vi "Variant-with-Array-Data-Type_to_String.vi"(8 "error in (no error)":errorcluster, 11 "variant":variant) -> (0 "error out":errorcluster, 3 "string":string)   [LabVIEW 2013]
doc: "Converts a variant, which contains an array element of almost any type, to a concatenated string where each value is separated by a space."
uses:
  <vilib>/Utility/VariantDataType/VariantType.lvlib
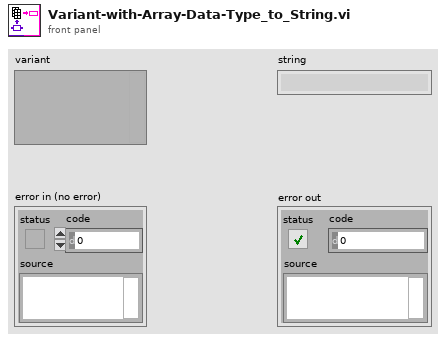
[diagram p1: front panel]
types:
  T1 = typedef "VariantType.lvlib/Type.ctl" = enum8{"Invalid Type", "Void", "I8", "I16", "I32", "I64", "U8", "U16", "U32", "U64", "Single Float", "Double Float", "Extended Float", "Single Complex", "Double Complex", "Extended Complex", "Enum U8", "Enum U16", "Enum U32", "Enum U64", "Single Float With Unit", "Double Float With Unit", "Extended Float With Unit", "Single Complex with Unit", "Double Complex with Unit", "Extended Complex with Unit", "Boolean", "String", "Path", "Picture", "Tag", "Array", "Cluster", "Variant", "LV Variant", "Waveform", "Timestamp", "Digital Waveform", "Digital Data", "ExpressData", "Refnum", "External Data", "VI", "Poly VI", "LabVIEW Class Instance", "Fixed Point"}
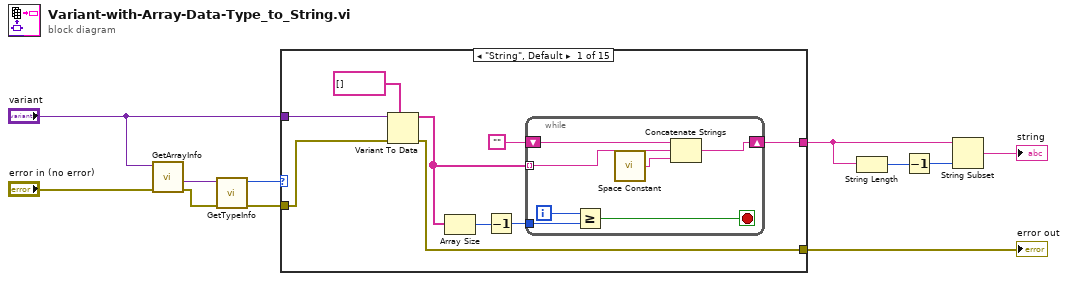
[diagram p0: block diagram]
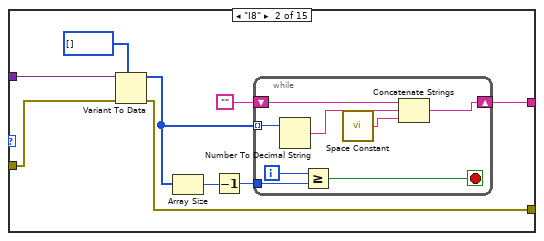
[diagram p2: hidden frame]
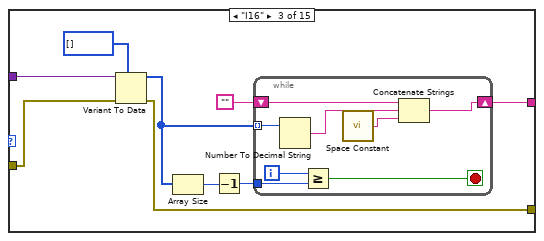
[diagram p3: hidden frame]
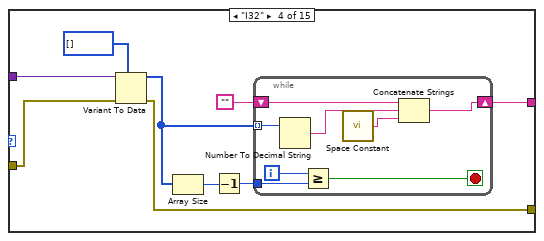
[diagram p4: hidden frame]
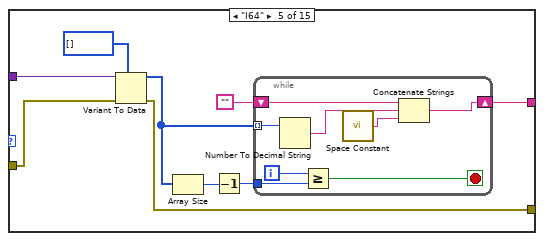
[diagram p5: hidden frame]
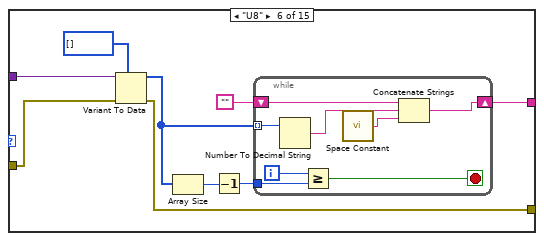
[diagram p6: hidden frame]
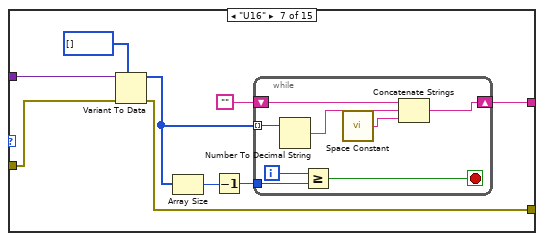
[diagram p7: hidden frame]
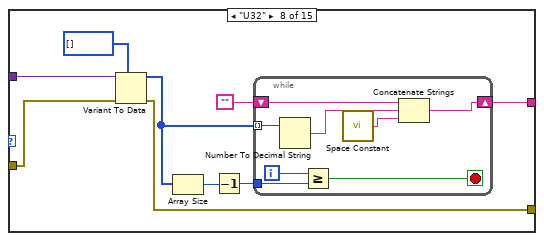
[diagram p8: hidden frame]
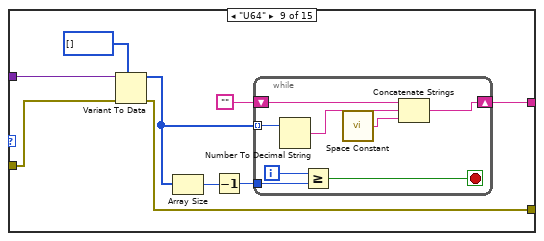
[diagram p9: hidden frame]
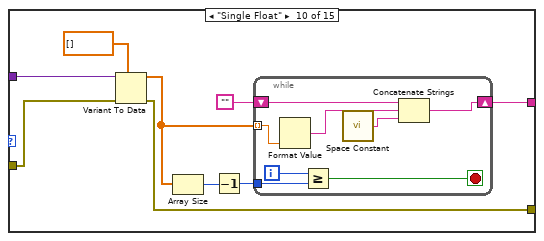
[diagram p10: hidden frame]
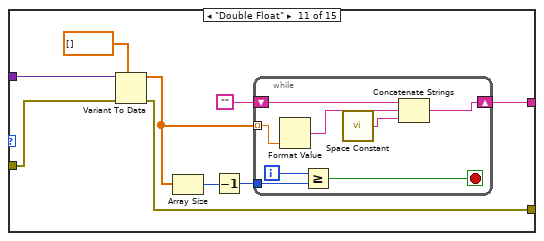
[diagram p11: hidden frame]
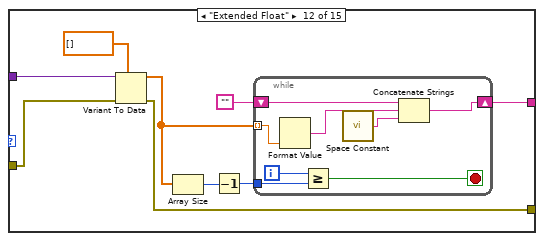
[diagram p12: hidden frame]
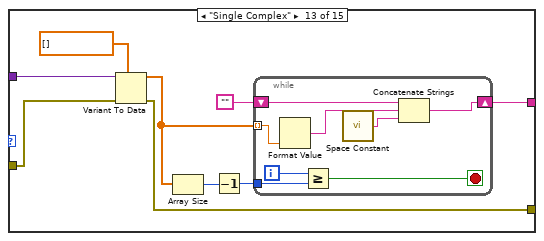
[diagram p13: hidden frame]
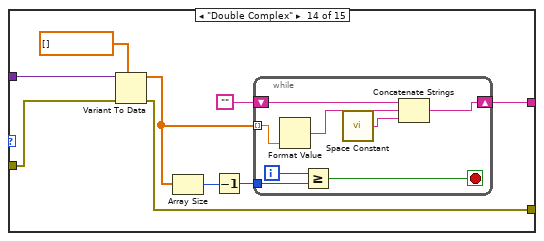
[diagram p14: hidden frame]
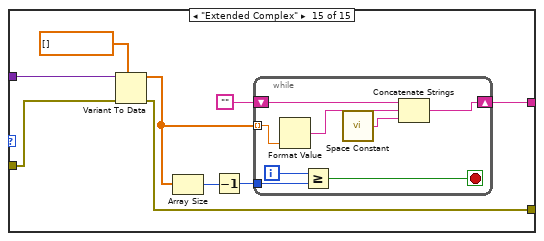
[diagram p15: hidden frame]
diagram:
  n1 = call <vilib>:"GetArrayInfo.vi"("error in (no error)"="error in (no error)", "Variant"="variant") -> ("error out"=w4:errorcluster, "ArrayElement"=w6:variant)  [unwired: 6 in, 2 out]
  n2 = call <vilib>:"GetTypeInfo.vi"("error in (no error)"=w4, "Variant"=w6) -> ("error out"=w3:errorcluster, "Type Enum"=w7:T1)  [unwired: 5 in, 3 out]
  n3 = case shown="\"String\", Default" w7 {
    tunnel: "variant" -> [w20 w36 w53 w70 w87 w104 w121 w138 w155 w172 w189 w206 w223 w240 w257]
    tunnel: [w15 w31 w48 w65 w82 w99 w116 w133 w150 w167 w184 w201 w218 w235 w252] -> w10
    tunnel: w3 -> [w13 w28 w45 w62 w79 w96 w113 w130 w147 w165 w181 w198 w215 w232 w249]
    tunnel: [w12 w29 w46 w63 w80 w97 w114 w131 w148 w164 w182 w199 w216 w233 w250] -> w2
    frame "String", Default {
      n4 = Variant To Data(error in=w13, type=string[] [], Variant=w20) -> (data=w17:string[], error out=w12:errorcluster)
      n5 = Array Size(array=w17) -> (size(s)=w19:i32)
      n6 = Decrement(x=w19) -> (x-1=w14:i32)
      n7 = while {
        tunnel: w17 -> [w21] mode=indexing
        shift-right: [w26] -> w15
        shift-left: "" -> [w27]
        tunnel: w14 -> [w22]
        i -> [w23]
        stop <- w24 stop-if-true
        n8 = Greater Or Equal?(x=w23, y=w22) -> (x >= y?=w24:bool)
        n9 = call <vilib>:"Space Constant.vi"() -> ("String"=w25:string)
        n10 = Concatenate Strings(w27, w21, w25) -> (w26:string)
      }
    }
    frame "I8" {
      n11 = Variant To Data(error in=w28, type=i8[] [], Variant=w36) -> (data=w33:i8[], error out=w29:errorcluster)
      n12 = Array Size(array=w33) -> (size(s)=w35:i32)
      n13 = Decrement(x=w35) -> (x-1=w30:i32)
      n14 = while {
        tunnel: w33 -> [w44] mode=indexing
        shift-right: [w42] -> w31
        shift-left: "" -> [w43]
        tunnel: w30 -> [w37]
        i -> [w38]
        stop <- w39 stop-if-true
        n15 = Number To Decimal String(number=w44) -> (decimal integer string=w41:string)  [unwired: 1 in]
        n16 = Greater Or Equal?(x=w38, y=w37) -> (x >= y?=w39:bool)
        n17 = call <vilib>:"Space Constant.vi"() -> ("String"=w40:string)
        n18 = Concatenate Strings(w43, w41, w40) -> (w42:string)
      }
    }
    frame "I16" {
      n19 = Variant To Data(error in=w45, type=i16[] [], Variant=w53) -> (data=w50:i16[], error out=w46:errorcluster)
      n20 = Array Size(array=w50) -> (size(s)=w52:i32)
      n21 = Decrement(x=w52) -> (x-1=w47:i32)
      n22 = while {
        tunnel: w50 -> [w61] mode=indexing
        shift-right: [w59] -> w48
        shift-left: "" -> [w60]
        tunnel: w47 -> [w54]
        i -> [w55]
        stop <- w56 stop-if-true
        n23 = Number To Decimal String(number=w61) -> (decimal integer string=w58:string)  [unwired: 1 in]
        n24 = Greater Or Equal?(x=w55, y=w54) -> (x >= y?=w56:bool)
        n25 = call <vilib>:"Space Constant.vi"() -> ("String"=w57:string)
        n26 = Concatenate Strings(w60, w58, w57) -> (w59:string)
      }
    }
    frame "I32" {
      n27 = Variant To Data(error in=w62, type=i32[] [], Variant=w70) -> (data=w67:i32[], error out=w63:errorcluster)
      n28 = Array Size(array=w67) -> (size(s)=w69:i32)
      n29 = Decrement(x=w69) -> (x-1=w64:i32)
      n30 = while {
        tunnel: w67 -> [w78] mode=indexing
        shift-right: [w76] -> w65
        shift-left: "" -> [w77]
        tunnel: w64 -> [w71]
        i -> [w72]
        stop <- w73 stop-if-true
        n31 = Number To Decimal String(number=w78) -> (decimal integer string=w75:string)  [unwired: 1 in]
        n32 = Greater Or Equal?(x=w72, y=w71) -> (x >= y?=w73:bool)
        n33 = call <vilib>:"Space Constant.vi"() -> ("String"=w74:string)
        n34 = Concatenate Strings(w77, w75, w74) -> (w76:string)
      }
    }
    frame "I64" {
      n35 = Variant To Data(error in=w79, type=i64[] [], Variant=w87) -> (data=w84:i64[], error out=w80:errorcluster)
      n36 = Array Size(array=w84) -> (size(s)=w86:i32)
      n37 = Decrement(x=w86) -> (x-1=w81:i32)
      n38 = while {
        tunnel: w84 -> [w95] mode=indexing
        shift-right: [w93] -> w82
        shift-left: "" -> [w94]
        tunnel: w81 -> [w88]
        i -> [w89]
        stop <- w90 stop-if-true
        n39 = Number To Decimal String(number=w95) -> (decimal integer string=w92:string)  [unwired: 1 in]
        n40 = Greater Or Equal?(x=w89, y=w88) -> (x >= y?=w90:bool)
        n41 = call <vilib>:"Space Constant.vi"() -> ("String"=w91:string)
        n42 = Concatenate Strings(w94, w92, w91) -> (w93:string)
      }
    }
    frame "U8" {
      n43 = Variant To Data(error in=w96, type=u8[] [], Variant=w104) -> (data=w101:u8[], error out=w97:errorcluster)
      n44 = Array Size(array=w101) -> (size(s)=w103:i32)
      n45 = Decrement(x=w103) -> (x-1=w98:i32)
      n46 = while {
        tunnel: w101 -> [w112] mode=indexing
        shift-right: [w110] -> w99
        shift-left: "" -> [w111]
        tunnel: w98 -> [w105]
        i -> [w106]
        stop <- w107 stop-if-true
        n47 = Number To Decimal String(number=w112) -> (decimal integer string=w109:string)  [unwired: 1 in]
        n48 = Greater Or Equal?(x=w106, y=w105) -> (x >= y?=w107:bool)
        n49 = call <vilib>:"Space Constant.vi"() -> ("String"=w108:string)
        n50 = Concatenate Strings(w111, w109, w108) -> (w110:string)
      }
    }
    frame "U16" {
      n51 = Variant To Data(error in=w113, type=u16[] [], Variant=w121) -> (data=w118:u16[], error out=w114:errorcluster)
      n52 = Array Size(array=w118) -> (size(s)=w120:i32)
      n53 = Decrement(x=w120) -> (x-1=w115:i32)
      n54 = while {
        tunnel: w118 -> [w129] mode=indexing
        shift-right: [w127] -> w116
        shift-left: "" -> [w128]
        tunnel: w115 -> [w122]
        i -> [w123]
        stop <- w124 stop-if-true
        n55 = Number To Decimal String(number=w129) -> (decimal integer string=w126:string)  [unwired: 1 in]
        n56 = Greater Or Equal?(x=w123, y=w122) -> (x >= y?=w124:bool)
        n57 = call <vilib>:"Space Constant.vi"() -> ("String"=w125:string)
        n58 = Concatenate Strings(w128, w126, w125) -> (w127:string)
      }
    }
    frame "U32" {
      n59 = Variant To Data(error in=w130, type=u32[] [], Variant=w138) -> (data=w135:u32[], error out=w131:errorcluster)
      n60 = Array Size(array=w135) -> (size(s)=w137:i32)
      n61 = Decrement(x=w137) -> (x-1=w132:i32)
      n62 = while {
        tunnel: w135 -> [w146] mode=indexing
        shift-right: [w144] -> w133
        shift-left: "" -> [w145]
        tunnel: w132 -> [w139]
        i -> [w140]
        stop <- w141 stop-if-true
        n63 = Number To Decimal String(number=w146) -> (decimal integer string=w143:string)  [unwired: 1 in]
        n64 = Greater Or Equal?(x=w140, y=w139) -> (x >= y?=w141:bool)
        n65 = call <vilib>:"Space Constant.vi"() -> ("String"=w142:string)
        n66 = Concatenate Strings(w145, w143, w142) -> (w144:string)
      }
    }
    frame "U64" {
      n67 = Variant To Data(error in=w147, type=u64[] [], Variant=w155) -> (data=w152:u64[], error out=w148:errorcluster)
      n68 = Array Size(array=w152) -> (size(s)=w154:i32)
      n69 = Decrement(x=w154) -> (x-1=w149:i32)
      n70 = while {
        tunnel: w152 -> [w163] mode=indexing
        shift-right: [w161] -> w150
        shift-left: "" -> [w162]
        tunnel: w149 -> [w156]
        i -> [w157]
        stop <- w158 stop-if-true
        n71 = Number To Decimal String(number=w163) -> (decimal integer string=w160:string)  [unwired: 1 in]
        n72 = Greater Or Equal?(x=w157, y=w156) -> (x >= y?=w158:bool)
        n73 = call <vilib>:"Space Constant.vi"() -> ("String"=w159:string)
        n74 = Concatenate Strings(w162, w160, w159) -> (w161:string)
      }
    }
    frame "Single Float" {
      n75 = Variant To Data(error in=w165, type=sgl[] [], Variant=w172) -> (data=w169:sgl[], error out=w164:errorcluster)
      n76 = Array Size(array=w169) -> (size(s)=w171:i32)
      n77 = Decrement(x=w171) -> (x-1=w166:i32)
      n78 = while {
        tunnel: w169 -> [w173] mode=indexing
        shift-right: [w179] -> w167
        shift-left: "" -> [w180]
        tunnel: w166 -> [w174]
        i -> [w175]
        stop <- w176 stop-if-true
        n79 = Format Value(value (0)=w173) -> (output string=w178:string)  [unwired: 2 in]
        n80 = Greater Or Equal?(x=w175, y=w174) -> (x >= y?=w176:bool)
        n81 = call <vilib>:"Space Constant.vi"() -> ("String"=w177:string)
        n82 = Concatenate Strings(w180, w178, w177) -> (w179:string)
      }
    }
    frame "Double Float" {
      n83 = Variant To Data(error in=w181, type=dbl[] [], Variant=w189) -> (data=w186:dbl[], error out=w182:errorcluster)
      n84 = Array Size(array=w186) -> (size(s)=w188:i32)
      n85 = Decrement(x=w188) -> (x-1=w183:i32)
      n86 = while {
        tunnel: w186 -> [w190] mode=indexing
        shift-right: [w196] -> w184
        shift-left: "" -> [w197]
        tunnel: w183 -> [w191]
        i -> [w192]
        stop <- w193 stop-if-true
        n87 = Format Value(value (0)=w190) -> (output string=w195:string)  [unwired: 2 in]
        n88 = Greater Or Equal?(x=w192, y=w191) -> (x >= y?=w193:bool)
        n89 = call <vilib>:"Space Constant.vi"() -> ("String"=w194:string)
        n90 = Concatenate Strings(w197, w195, w194) -> (w196:string)
      }
    }
    frame "Extended Float" {
      n91 = Variant To Data(error in=w198, type=ext[] [], Variant=w206) -> (data=w203:ext[], error out=w199:errorcluster)
      n92 = Array Size(array=w203) -> (size(s)=w205:i32)
      n93 = Decrement(x=w205) -> (x-1=w200:i32)
      n94 = while {
        tunnel: w203 -> [w207] mode=indexing
        shift-right: [w213] -> w201
        shift-left: "" -> [w214]
        tunnel: w200 -> [w208]
        i -> [w209]
        stop <- w210 stop-if-true
        n95 = Format Value(value (0)=w207) -> (output string=w212:string)  [unwired: 2 in]
        n96 = Greater Or Equal?(x=w209, y=w208) -> (x >= y?=w210:bool)
        n97 = call <vilib>:"Space Constant.vi"() -> ("String"=w211:string)
        n98 = Concatenate Strings(w214, w212, w211) -> (w213:string)
      }
    }
    frame "Single Complex" {
      n99 = Variant To Data(error in=w215, type=csg[] [], Variant=w223) -> (data=w220:csg[], error out=w216:errorcluster)
      n100 = Array Size(array=w220) -> (size(s)=w222:i32)
      n101 = Decrement(x=w222) -> (x-1=w217:i32)
      n102 = while {
        tunnel: w220 -> [w224] mode=indexing
        shift-right: [w230] -> w218
        shift-left: "" -> [w231]
        tunnel: w217 -> [w225]
        i -> [w226]
        stop <- w227 stop-if-true
        n103 = Format Value(value (0)=w224) -> (output string=w229:string)  [unwired: 2 in]
        n104 = Greater Or Equal?(x=w226, y=w225) -> (x >= y?=w227:bool)
        n105 = call <vilib>:"Space Constant.vi"() -> ("String"=w228:string)
        n106 = Concatenate Strings(w231, w229, w228) -> (w230:string)
      }
    }
    frame "Double Complex" {
      n107 = Variant To Data(error in=w232, type=cdb[] [], Variant=w240) -> (data=w237:cdb[], error out=w233:errorcluster)
      n108 = Array Size(array=w237) -> (size(s)=w239:i32)
      n109 = Decrement(x=w239) -> (x-1=w234:i32)
      n110 = while {
        tunnel: w237 -> [w241] mode=indexing
        shift-right: [w247] -> w235
        shift-left: "" -> [w248]
        tunnel: w234 -> [w242]
        i -> [w243]
        stop <- w244 stop-if-true
        n111 = Format Value(value (0)=w241) -> (output string=w246:string)  [unwired: 2 in]
        n112 = Greater Or Equal?(x=w243, y=w242) -> (x >= y?=w244:bool)
        n113 = call <vilib>:"Space Constant.vi"() -> ("String"=w245:string)
        n114 = Concatenate Strings(w248, w246, w245) -> (w247:string)
      }
    }
    frame "Extended Complex" {
      n115 = Variant To Data(error in=w249, type=cxt[] [], Variant=w257) -> (data=w254:cxt[], error out=w250:errorcluster)
      n116 = Array Size(array=w254) -> (size(s)=w256:i32)
      n117 = Decrement(x=w256) -> (x-1=w251:i32)
      n118 = while {
        tunnel: w254 -> [w258] mode=indexing
        shift-right: [w264] -> w252
        shift-left: "" -> [w265]
        tunnel: w251 -> [w259]
        i -> [w260]
        stop <- w261 stop-if-true
        n119 = Format Value(value (0)=w258) -> (output string=w263:string)  [unwired: 2 in]
        n120 = Greater Or Equal?(x=w260, y=w259) -> (x >= y?=w261:bool)
        n121 = call <vilib>:"Space Constant.vi"() -> ("String"=w262:string)
        n122 = Concatenate Strings(w265, w263, w262) -> (w264:string)
      }
    }
  }
  "error out" <- w2
  n123 = String Length(string=w10) -> (length=w8:i32)
  n124 = Decrement(x=w8) -> (x-1=w9:i32)
  n125 = String Subset(string=w10, length (rest)=w9) -> (substring=→"string":string)  [unwired: 1 in]
